vi "Immediate Measure.vi"(7 "Restore Range?(T)":bool=TRUE, 8 "error in (no error)":errorcluster, 9 "Max Time (-1ms)":i32=-1, 10 "Measurements to Acquire(1)":i32=1 min=0, 11 "DMM Driver in":refnum<class "DMM Driver.lvclass">) -> (0 "error out":errorcluster, 1 "Function":T2, 2 "Measurements":dbl[](array[numeric]), 3 "DMM Driver out":refnum<class "DMM Driver.lvclass">, 4 "Range":dbl, 5 "Digit Resolution(5½)":T1=enum."5½")   [LabVIEW 2020, in "DMM.lvlib" / "DMM Driver.lvclass"]
doc: "Perform a measurement operation on the DMM.\nThe measurements are returned together with the current configuration of the DMM.\nIf needed the DMM will autorange before performing the measurements. The DMM range is restored after the measurements."
uses:
  DMM Driver.lvclass
  Controls/Ctl_DigitResolution.ctl
  DMM.lvlib
  Controls/Ctl_Function.ctl
  Controls/Community/Ctl_Config.ctl
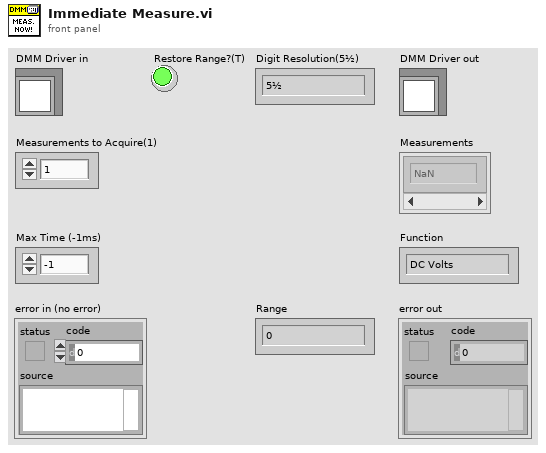
[diagram p1: front panel]
types:
  T1 = typedef "DMM.lvlib/Ctl_DigitResolution.ctl" = enum8{"3½", "4½", "5½", "6½", "7½"}
  T2 = typedef "DMM.lvlib/Ctl_Function.ctl" = enum8{"DC Volts", "AC Volts", "DC Current", "AC Current", "2-wire Resistance", "4-wire Resistance", "Diode", "Frequency", "Period", "AC Volts DC Coupled", "Capacitance", "Inductance", "Temperature"}
  T3 = typedef "DMM.lvlib/Ctl_Config.ctl" = cluster{"Function":T2, "Range":dbl, "Digit Resolution(5½)":T1}
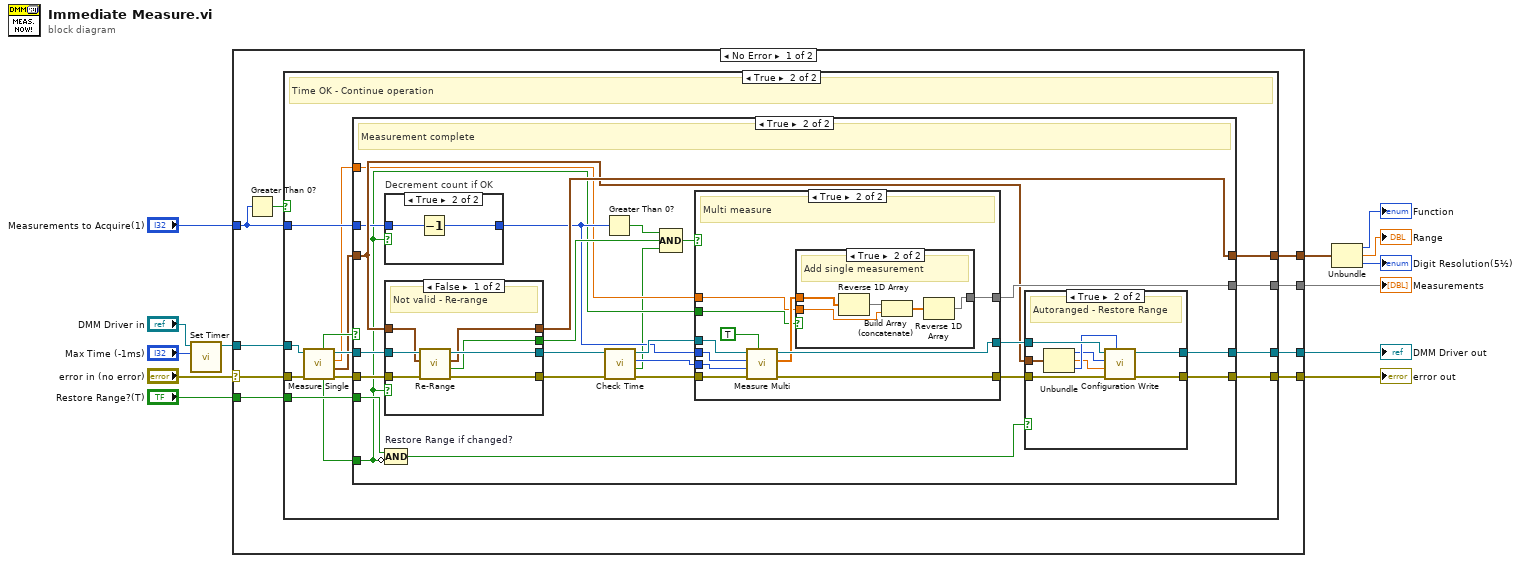
[diagram p0: block diagram]
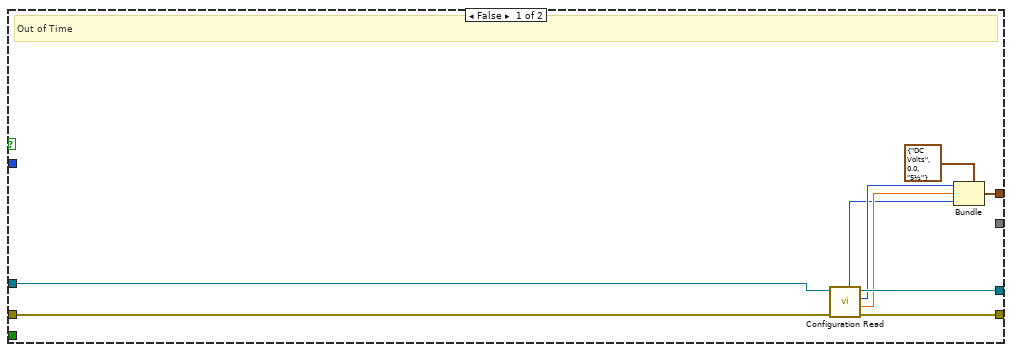
[diagram p2: hidden frame]
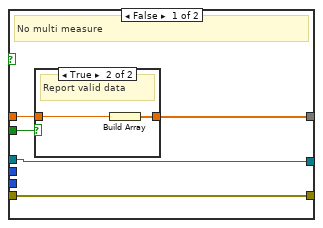
[diagram p6: hidden frame]
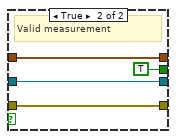
[diagram p9: hidden frame]
diagram:
  n1 = call "Set Timer.vi"("Max Time (-1ms)"="Max Time (-1ms)", "DMM Driver in"="DMM Driver in") -> ("DMM Driver out"=w9:refnum<class "DMM Driver.lvclass">)  [unwired: 9 in]
  n2 = case shown="No Error" "error in (no error)" {
    selector: "error in (no error)" -> [w21 w122]
    tunnel: [w17 w122] -> w12
    tunnel: [w20 w121] -> w10
    tunnel: w9 -> [w22 w121]
    tunnel: "Measurements to Acquire(1)" -> [w19 _]
    tunnel: [w18 _] -> w5
    tunnel: [w16 _] -> w6
    tunnel: "Restore Range?(T)" -> [w15 _]
    frame No Error {
      n3 = Greater Than 0?(x=w19) -> (x > 0?=w14:bool)
      n4 = case shown="True" w14 {
        tunnel: w22 -> [w31 w39]
        tunnel: w21 -> [w29 w35]
        tunnel: [w28 w45] -> w17
        tunnel: [w30 w44] -> w20
        tunnel: w19 -> [_ w43]
        tunnel: [_ w42] -> w18
        tunnel: [w24 w41] -> w16
        tunnel: w15 -> [_ w40]
        frame False {
          # "Out of Time"
          n5 = call-dynamic "Configuration Read.vi"("error in (no error)"=w29, "DMM Driver in"=w31) -> ("error out"=w28:errorcluster, "Range"=w27:dbl, "Function"=w26:T2, "DMM Driver out"=w30:refnum<class "DMM Driver.lvclass">, "Digit Resolution(5½)"=w25:T1)  [unwired: 5 in]
          n6 = Bundle(cluster=T3 {"Function"=enum."DC Volts", "Range"=0.0, "Digit Resolution(5½)"=enum."5½"} ("Config"), "Function"=w26, "Range"=w27, "Digit Resolution(5½)"=w25) -> (w24:T3)
        }
        frame True {
          # "Time OK - Continue operation"
          n7 = call "Measure Single.vi"("error in (no error)"=w35, "DMM Driver in"=w39) -> ("error out"=w32:errorcluster, "Config"=w34:T3, "Measurement"=w33:dbl, "DMM Driver out"=w38:refnum<class "DMM Driver.lvclass">, "Valid measurement?"=w36:bool, "Finished?"=w37:bool)  [unwired: 4 in]
          n8 = case shown="True" w37 {
            tunnel: w36 -> [_ w51]
            tunnel: [w47 w66] -> w45
            tunnel: w32 -> [w47 w58]
            tunnel: [w48 w64] -> w44
            tunnel: w38 -> [w48 w59]
            tunnel: w33 -> [_ w53]
            tunnel: w43 -> [_ w55]
            tunnel: [_ w62] -> w42
            tunnel: [w46 w61] -> w41
            tunnel: w34 -> [w46 w60]
            tunnel: w40 -> [_ w52]
            frame False {
              # "Out of Time"
            }
            frame True {
              # "Measurement complete"
              n9 = case "Decrement count if OK" shown="True" w51 {
                tunnel: w55 -> [w83 w85]
                tunnel: [w83 w84] -> w54
                frame False {
                }
                frame True {
                  n10 = Decrement(x=w85) -> (x-1=w84:i32)
                }
              }
              n11 = case shown="False" w51 {
                tunnel: [w116 w120] -> w71
                tunnel: w58 -> [w112 w120]
                tunnel: [w115 w119] -> w72
                tunnel: w59 -> [w113 w119]
                tunnel: [w114 TRUE ("Success?")] -> w57
                tunnel: [w110 w117] -> w61
                tunnel: w60 -> [w111 w117]
                frame False {
                  # "Not valid - Re-range"
                  n12 = call "Re-Range.vi"("error in (no error)"=w112, "Config in"=w111, "DMM Driver in"=w113) -> ("error out"=w116:errorcluster, "Success?"=w114:bool, "Config out"=w110:T3, "DMM Driver out"=w115:refnum<class "DMM Driver.lvclass">)  [unwired: 5 in]
                }
                frame True {
                  # "Valid measurement"
                }
              }
              n13 = Compound Arithmetic op=AND "Restore Range if changed?"(w52, invert w51) -> (w50:bool)
              n14 = Greater Than 0?(x=w54) -> (x > 0?=w56:bool)
              n15 = call "Check Time.vi"("error in (no error)"=w71, "DMM Driver in"=w72) -> ("error out"=w69:errorcluster, "Time OK?"=w49:bool, "Remaining Time"=w67:i32, "DMM Driver out"=w68:refnum<class "DMM Driver.lvclass">)  [unwired: 6 in]
              n16 = Compound Arithmetic op=AND(w56, w57, w49) -> (w70:bool)
              n17 = case shown="True" w70 {
                tunnel: w69 -> [w89 w102]
                tunnel: w54 -> [_ w94]
                tunnel: [w90 w99] -> w63
                tunnel: w68 -> [w90 w101]
                tunnel: [w89 w100] -> w65
                tunnel: w67 -> [_ w103]
                tunnel: w53 -> [w87 w96]
                tunnel: [w86 w97] -> w62
                tunnel: w51 -> [w88 w95]
                frame False {
                  # "No multi measure"
                  n18 = case shown="True" w88 {
                    tunnel: w87 -> [_ w92]
                    tunnel: [_ w91] -> w86
                    frame False {
                      # "No valid data"
                    }
                    frame True {
                      # "Report valid data"
                      n19 = Build Array(w92) -> (w91:dbl[])
                    }
                  }
                }
                frame True {
                  # "Multi measure"
                  n20 = call-dynamic "Measure Multi.vi"("Config for Immediate Measure?(T)"=TRUE, "error in (no error)"=w102, "Max Time (-1ms)"=w103, "Measurements to Acquire(1)"=w94, "DMM Driver in"=w101) -> ("error out"=w100:errorcluster, "Measurements"=w98:dbl[], "DMM Driver out"=w99:refnum<class "DMM Driver.lvclass">)  [unwired: 4 in]
                  n21 = case shown="True" w95 {
                    tunnel: w98 -> [w104 w109]
                    tunnel: [w104 w105] -> w97
                    tunnel: w96 -> [_ w107]
                    frame False {
                    }
                    frame True {
                      # "Add single measurement"
                      n22 = Reverse 1D Array(array=w109) -> (reversed array=w108:dbl[])
                      n23 = Build Array (concatenate)(w108, w107) -> (w106:dbl[])
                      n24 = Reverse 1D Array(array=w106) -> (reversed array=w105:dbl[])
                    }
                  }
                }
              }
              n25 = case "Restore Range if changed?" shown="True" w50 {
                tunnel: [w74 w75] -> w66
                tunnel: w65 -> [w74 w76]
                tunnel: [w73 w80] -> w64
                tunnel: w63 -> [w73 w81]
                tunnel: w60 -> [_ w82]
                frame False {
                }
                frame True {
                  # "Autoranged - Restore Range"
                  n26 = Unbundle(w82) -> ("Function"=w78:T2, "Range"=w77:dbl, "Digit Resolution(5½)"=w79:T1)
                  n27 = call "Configuration Write.vi"("Digit Resolution(5½)"=w79, "error in (no error)"=w76, "Range"=w77, "Function"=w78, "DMM Driver in"=w81) -> ("error out"=w75:errorcluster, "DMM Driver out"=w80:refnum<class "DMM Driver.lvclass">)  [unwired: 4 in, 1 out]
                }
              }
            }
          }
        }
      }
    }
    frame Error {
    }
  }
  "error out" <- w12
  "DMM Driver out" <- w10
  "Measurements" <- w5
  n28 = Unbundle(w6) -> ("Function"=→"Function":T2, "Range"=→"Range":dbl, "Digit Resolution(5½)"=→"Digit Resolution(5½)":T1)
